vi "ui_globals.vi"() -> ()   [LabVIEW 2013]
panel:
  in  "Override VIs":string[](array[string])
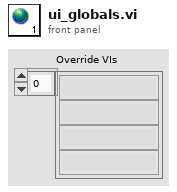
[diagram p1: front panel]
diagram:
